vi "DoPictureSplit.vi"(8 "SmallSquarewidth(Y)":i32, 9 "SmallSquarelength(X)":i32, 10 "image data":T1, 11 "NxN to Split":i32) -> (2 "2D picture array":picture[][](array[picture]))   [LabVIEW 2014]
uses:
  <vilib>/picture/picture.llb/imagedata.ctl
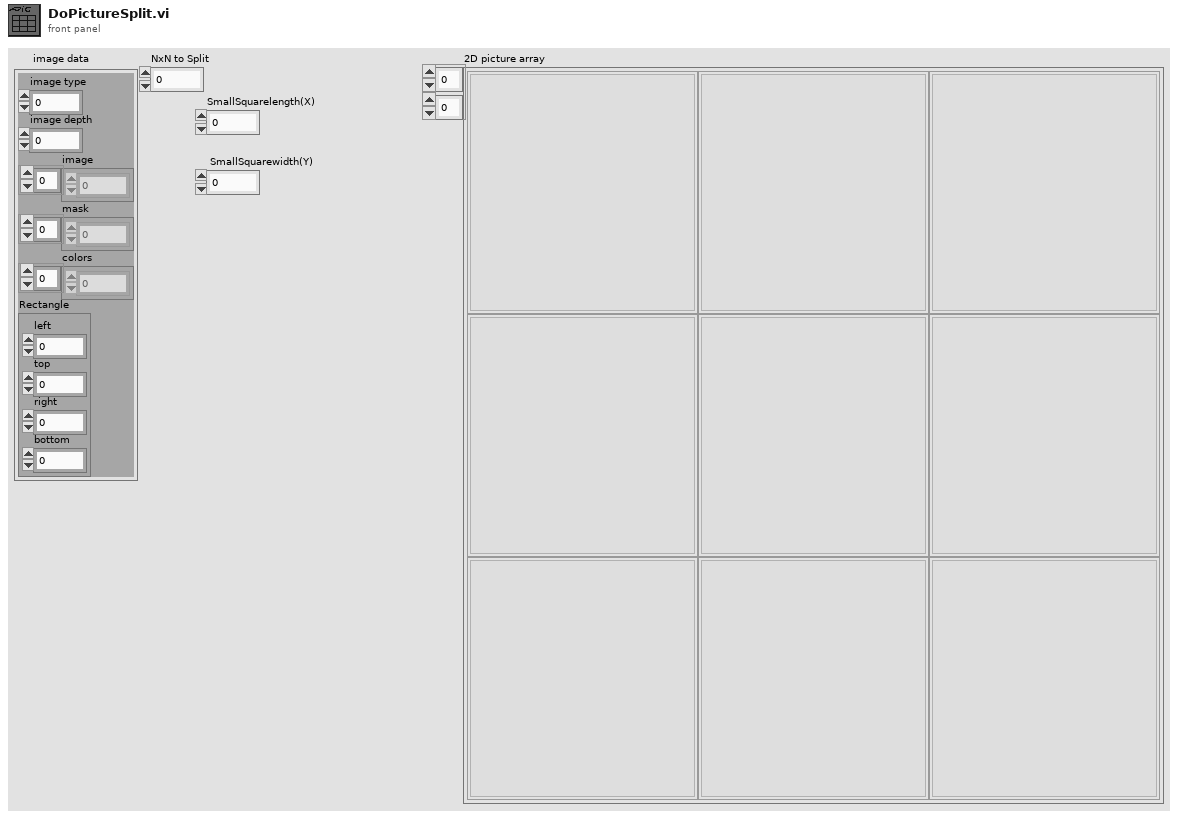
[diagram p1: front panel]
types:
  T1 = typedef "imagedata.ctl" = cluster{"image type":i32, "image depth":i32, "image":u8[], "mask":u8[], "colors":u32[], "Rectangle":cluster{"left":i16, "top":i16, "right":i16, "bottom":i16}}
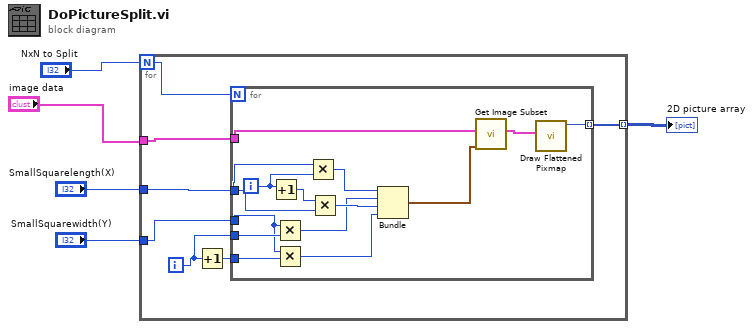
[diagram p0: block diagram]
diagram:
  n1 = for {
    N: "NxN to Split" -> [w11]
    tunnel: "image data" -> [w12]
    tunnel: "SmallSquarelength(X)" -> [w10]
    tunnel: "SmallSquarewidth(Y)" -> [w7]
    tunnel: [w6] -> w2 mode=indexing
    i -> [w8]
    n2 = Increment(x=w8) -> (x+1=w9:i32)
    n3 = for {
      N: w11 -> [_]
      tunnel: w12 -> [w25]
      tunnel: w10 -> [w13]
      tunnel: w9 -> [w20]
      tunnel: w8 -> [w19]
      tunnel: w7 -> [w18]
      tunnel: [w14] -> w6 mode=indexing
      i -> [w24]
      n4 = Increment(x=w24) -> (x+1=w22:i32)
      n5 = Multiply(x=w18, y=w19) -> (x*y=w17:i32)
      n6 = Multiply(x=w18, y=w20) -> (x*y=w16:i32)
      n7 = Multiply(x=w13, y=w24) -> (x*y=w23:i32)
      n8 = Multiply(x=w22, y=w13) -> (x*y=w21:i32)
      n9 = Bundle(w23, w17, w21, w16) -> (w15:cluster{i32, i32, i32, i32})  [unwired: 1 in]
      n10 = call <vilib>:"Get Image Subset.vi"("subset rect"=w15, "image data"=w25) -> ("image subset"=w26:T1)  [unwired: 4 in, 1 out]
      n11 = call <vilib>:"Draw Flattened Pixmap.vi"("image data"=w26) -> ("new picture"=w14:picture)  [unwired: 8 in]
    }
  }
  "2D picture array" <- w2
